vi "msgsBuilder_LaserScan.vi"(1 "intensities":dbl[](array[numeric]), 2 "ranges":dbl[](array[numeric]), 4 "range_max":sgl, 5 "range_min":sgl, 6 "scan_time":sgl, 7 "time_increment":sgl, 8 "angle_increment":sgl, 9 "angle_max":sgl, 10 "angle_min":sgl, 11 "msg in":string) -> (3 "sensor_msgs/LaserScan Out":string)   [LabVIEW 2016]
uses:
  <userlib>/ROS for LabVIEW Software/ROS/MessageBuilding/std_msgs/subs/float32Scalar.vi
  <userlib>/ROS for LabVIEW Software/ROS/MessageBuilding/std_msgs/subs/float32Array.vi
panel:
  in  "reset seq?":bool
  in  "frame_id":string
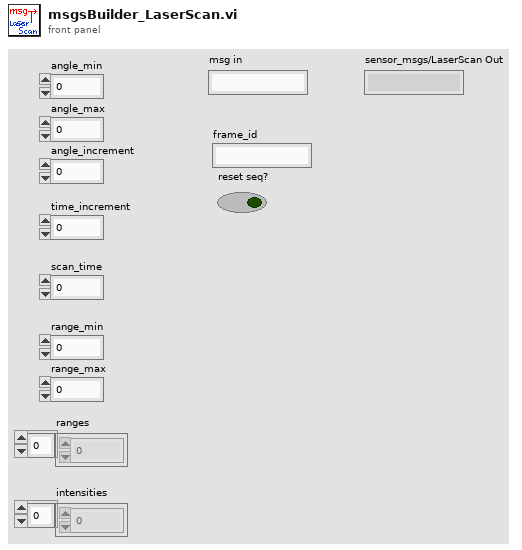
[diagram p1: front panel]
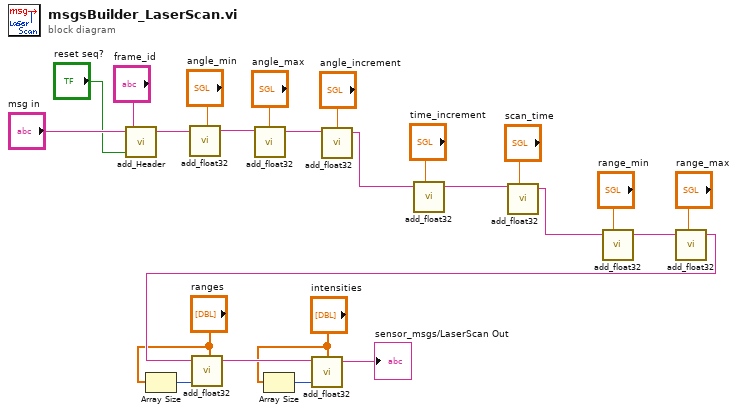
[diagram p0: block diagram]
diagram:
  n1 = call <userlib>:"add_Header.vi"("reset seq?"="reset seq?", "frame_id"="frame_id", "msg in"="msg in") -> ("msg out"=w11:string)  [unwired: 2 in]
  n2 = Array Size(array="ranges") -> (size(s)=w6:i32)
  n3 = call-poly <userlib>:"add_float32.vi"("Numeric"="angle_min", "msg in"=w11) -> ("msg out"=w17:string)  [unwired: 3 in]
  n4 = call-poly <userlib>:"add_float32.vi"("Numeric"="angle_max", "msg in"=w17) -> ("msg out"=w16:string)  [unwired: 3 in]
  n5 = Array Size(array="intensities") -> (size(s)=w4:i32)
  n6 = call-poly <userlib>:"add_float32.vi"("Numeric"="angle_increment", "msg in"=w16) -> ("msg out"=w15:string)  [unwired: 3 in]
  n7 = call-poly <userlib>:"add_float32.vi"("Numeric"="time_increment", "msg in"=w15) -> ("msg out"=w18:string)  [unwired: 3 in]
  n8 = call-poly <userlib>:"add_float32.vi"("Numeric"="scan_time", "msg in"=w18) -> ("msg out"=w13:string)  [unwired: 3 in]
  n9 = call-poly <userlib>:"add_float32.vi"("Numeric"="range_min", "msg in"=w13) -> ("msg out"=w12:string)  [unwired: 3 in]
  n10 = call-poly <userlib>:"add_float32.vi"("Numeric"="range_max", "msg in"=w12) -> ("msg out"=w10:string)  [unwired: 3 in]
  n11 = call-poly <userlib>:"add_float32.vi"("Array Length"=w6, "Array"="ranges", "msg in"=w10) -> ("msg out"=w8:string)  [unwired: 2 in]
  n12 = call-poly <userlib>:"add_float32.vi"("Array Length"=w4, "Array"="intensities", "msg in"=w8) -> ("msg out"=→"sensor_msgs/LaserScan Out":string)  [unwired: 2 in]
